vi "Buy Stock.vi"(11 "Stock Name":string) -> (3 "Response":string)   [LabVIEW 2020, in "Full Featured MCP Server.lvlib"]
uses:
  Full Featured MCP Server.lvlib
panel:
  out "error out":errorcluster
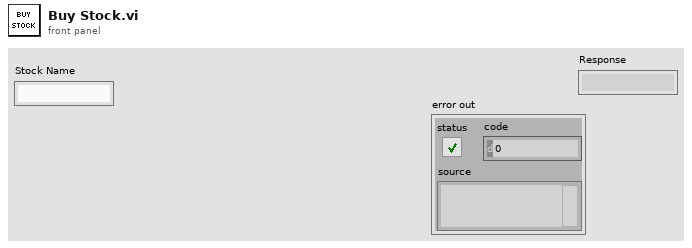
[diagram p1: front panel]
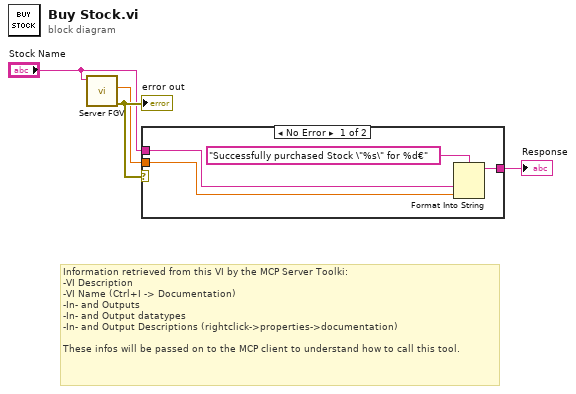
[diagram p0: block diagram]
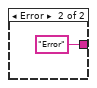
[diagram p2: hidden frame]
diagram:
  # "Information retrieved from this VI by the MCP Server Toolki:\n-VI Description\n-VI Name (Ctrl+I -> Documentation)\n-In- and Outputs\n-In- and Output datatypes\n-In- and Output Descriptions (rightclick->properties->documentation)\n\nThese infos will be passed on to the MCP client to understand how to call this tool."
  n1 = call "Server FGV.vi"("Stock Name"="Stock Name") -> ("error out"=w4:errorcluster, "purchase price"=w1:dbl)  [unwired: 8 in, 1 out]
  "error out" <- w4
  n2 = case shown="No Error" w4 {
    tunnel: [w7 "Error"] -> w3
    tunnel: "Stock Name" -> [w6 _]
    tunnel: w1 -> [w5 _]
    frame No Error {
      n3 = Format Into String(format string="Successfully purchased Stock \"%s\" for %d€", w6, w5) -> (resulting string=w7:string)  [unwired: 2 in, 1 out]
    }
    frame Error {
    }
  }
  "Response" <- w3
